vi "Acquire and logging.vi"() -> ()   [LabVIEW 2016]
uses:
  <vilib>/LabVIEW Interface for Arduino/Type Defs/Board Type.ctl
  <vilib>/LabVIEW Interface for Arduino/LabVIEW Interface for Arduino.lvlib
panel:
  out "error out 2":errorcluster
  out "Raw Data":dbl[](graph)
  in  "Analog Input Pin":u8
  out "Vout to save":dbl[](graph)
  in  "Acquition Speed":u32
  in  "Filename":path=path "D:/do an nang cao/data.xlsx"
  in  "Gain":dbl=99.0 format="%#_13g"
  out "error out":errorcluster
  in  "VISA resource":refnum<visa-resource-name>
  in  "stop":bool
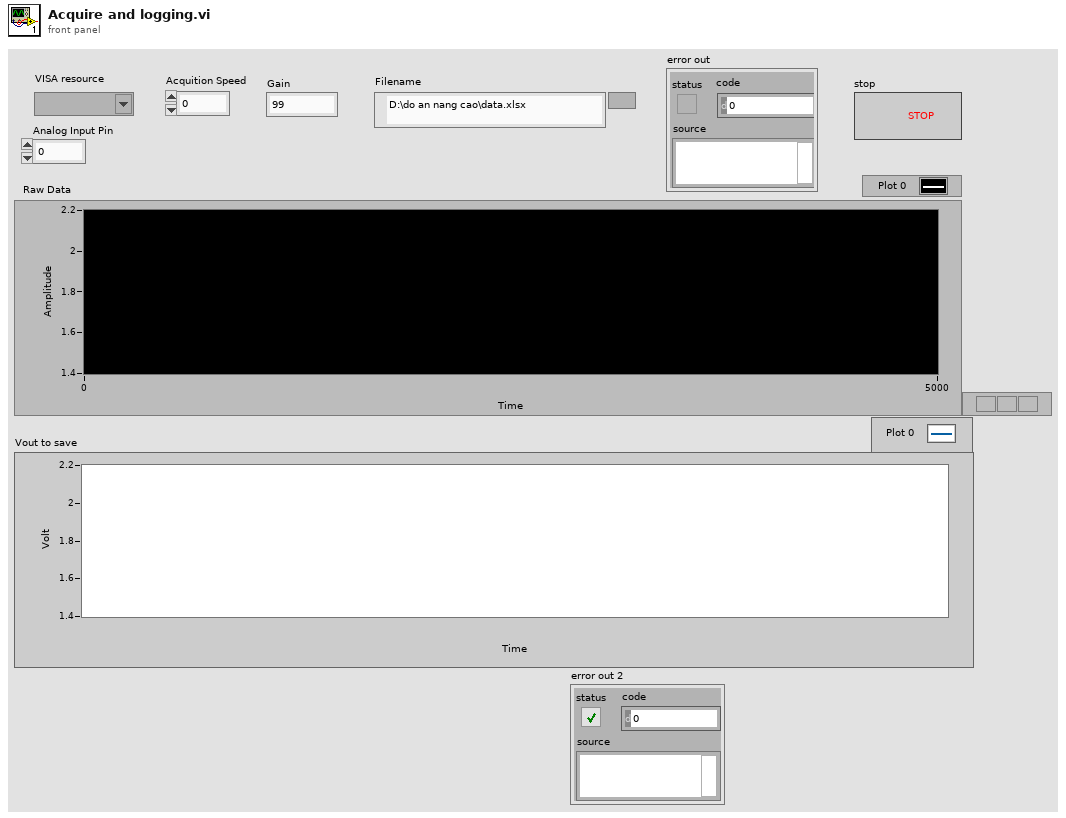
[diagram p1: front panel]
types:
  T1 = typedef "LabVIEW Interface for Arduino.lvlib/Board Type.ctl" = enum16{"Uno", "Dimuelanove w/Atmega 328", "Mega 2560"}
  T2 = typedef "LabVIEW Interface for Arduino.lvlib/Arduino Resource.ctl" = cluster{"VISA resource":refnum<visa-resource-name>, "Board Type":T1, "Connection Type":enum8{"USB / Serial"}, "Bytes Per Packet (15)":u8}
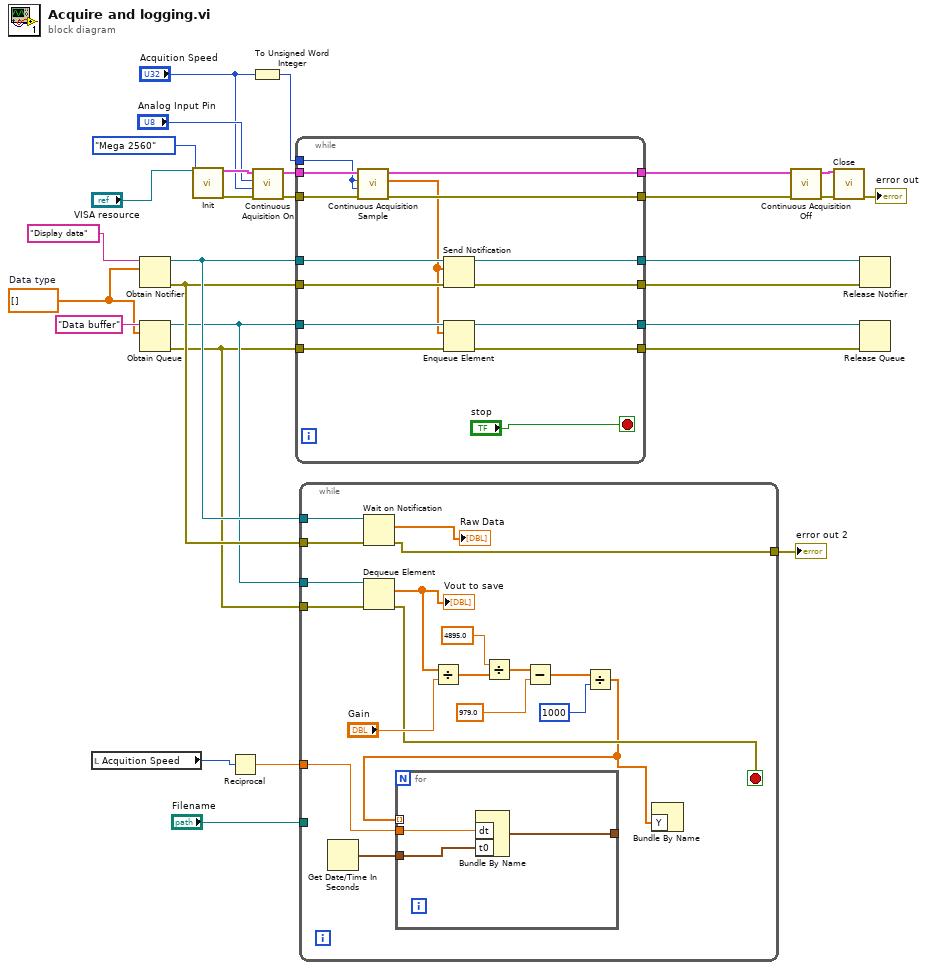
[diagram p0: block diagram]
diagram:
  w13 = dbl[] []  # Data type
  n1 = local read "Acquition Speed"() -> (w2:u32)
  n2 = Obtain Notifier(name (unnamed)="Display data", notification data type=w13) -> (notifier out=w10:refnum<notifier>, error out=w9:errorcluster)  [unwired: 2 in, 1 out]
  n3 = Obtain Queue(name (unnamed)="Data buffer", element data type=w13) -> (queue out=w8:refnum<queue>, error out=w7:errorcluster)  [unwired: 3 in, 1 out]
  n4 = call <vilib>:"Init.vi"("VISA resource"="VISA resource", "Board Type (Uno)"=Board_Type."Mega 2560") -> ("Arduino Resource"=w29:T2, "error out"=w25:errorcluster)  [unwired: 16 in]
  n5 = Reciprocal(x=w2) -> (1/x=w1:dbl)
  n6 = To Unsigned Word Integer(number="Acquition Speed") -> (unsigned 16bit integer=w19:u16)
  n7 = call <vilib>:"Continuous Aquisition On.vi"("error in"=w25, "Acquition Speed"="Acquition Speed", "Analog Input Pin"="Analog Input Pin", "Arduino Resource"=w29) -> ("error out"=w24:errorcluster, "Arduino Resource"=w28:T2)  [unwired: 6 in]
  n8 = while {
    tunnel: w28 -> [w44]
    tunnel: [w43] -> w27
    tunnel: w24 -> [w42]
    tunnel: [w41] -> w23
    tunnel: w19 -> [w39]
    tunnel: w10 -> [w38]
    tunnel: w9 -> [w37]
    tunnel: [w36] -> w15
    tunnel: [w35] -> w5
    tunnel: w8 -> [w34]
    tunnel: [w33] -> w12
    tunnel: [w32] -> w11
    tunnel: w7 -> [w31]
    stop <- "stop" stop-if-true
    n9 = call <vilib>:"Continuous Acquisition Sample.vi"("Arduino Resource"=w44, "Samples to Read"=w39, "Sample Rate (HZ)"=w39, "error in (no error)"=w42) -> ("Arduino Resource"=w43:T2, "Data"=w30:dbl[], "error out"=w41:errorcluster)  [unwired: 4 in]
    n10 = Send Notification(notification=w30, notifier=w38, error in (no error)=w37) -> (notifier out=w36:refnum<notifier>, error out=w35:errorcluster)
    n11 = Enqueue Element(queue=w34, element=w30, error in (no error)=w31) -> (queue out=w33:refnum<queue>, error out=w32:errorcluster)  [unwired: 1 in, 1 out]
  }
  n12 = while {
    tunnel: w10 -> [w62]
    tunnel: w9 -> [w61]
    tunnel: w8 -> [w59]
    tunnel: w7 -> [w58]
    tunnel: [w57] -> w4
    tunnel: "Filename" -> [_]
    tunnel: w1 -> [w46]
    stop <- w48 stop-if-true
    n13 = Get Date/Time In Seconds() -> (seconds since 1Jan1904=w47:timestamp)
    n14 = Wait on Notification(notifier=w62, error in (no error)=w61) -> (notification=→"Raw Data":dbl[], error out=w57:errorcluster)  [unwired: 2 in, 2 out]
    n15 = Dequeue Element(queue=w59, error in (no error)=w58) -> (element=w49:dbl[], error out=w48:errorcluster)  [unwired: 1 in, 2 out]
    "Vout to save" <- w49
    n16 = Divide(x=w49, y="Gain") -> (x/y=w51:dbl[])
    n17 = Divide(x=4895.0, y=w51) -> (x/y=w53:dbl[])
    n18 = Subtract(x=w53, y=979.0 ("x")) -> (x-y=w55:dbl[])
    n19 = Divide(x=w55, y=1000) -> (x/y=w45:dbl[])
    n20 = for {
      tunnel: w45 -> [_] mode=indexing
      tunnel: w47 -> [w65]
      tunnel: w46 -> [w64]
      tunnel: [w63] -> _
      n21 = Bundle By Name("dt"=w64, "t0"=w65) -> (w63:waveform(dbl))  [unwired: 1 in]
    }
    n22 = Bundle By Name("Y"=w45) -> ()  [unwired: 1 in, 1 out]
  }
  "error out 2" <- w4
  n23 = call <vilib>:"Continuous Acquisition Off.vi"("error in"=w23, "Arduino Resource"=w27) -> ("error out"=w22:errorcluster, "Arduino Resource"=w26:T2)  [unwired: 8 in]
  n24 = call <vilib>:"Close.vi"("Arduino Resource"=w26, "error in"=w22) -> ("error out"=→"error out":errorcluster)  [unwired: 13 in]
  n25 = Release Notifier(notifier=w15, error in (no error)=w5) -> ()  [unwired: 1 in, 3 out]
  n26 = Release Queue(queue=w12, error in (no error)=w11) -> ()  [unwired: 1 in, 3 out]
